vi "Refresh Default Value.vi"(8 "error in (no error)":errorcluster, 10 "Label":T1, 11 "Param Ref in":T5 format="%.0x") -> (0 "error out":errorcluster, 3 "Param Ref out":T5 format="%.0x")   [LabVIEW 2012, in "AIT 429 System Explorer.lvlib"]
uses:
  AIT 429 System Explorer.lvlib
  <vilib>/NI Veristand/Custom Device API/Custom Device Item Ref.ctl
  Controls/AIT_Label.ctl
  Controls/AIT_Word.ctl
  Controls/ARINCParam.ctl
  Shared/Controls and Global/TransferType.ctl
  <vilib>/NI Veristand/Custom Device Tools/Custom Device Utility Library/NI VeriStand - Search for All Items by GUID.vi
  Shared/Controls and Global/Global.vi
  <vilib>/NI Veristand/Custom Device API/Get Item Property (Double).vi
  <vilib>/NI Veristand/Custom Device API/Get Item Property (I32).vi
  <vilib>/NI Veristand/Custom Device API/Get Item Property (Boolean).vi
  ARINC 429 Shared.lvlib
  <vilib>/NI Veristand/Custom Device API/Custom Device API.lvlib
  <vilib>/NI Veristand/Custom Device Tools/Custom Device Utility Library/Custom Device Utility Library.lvlib
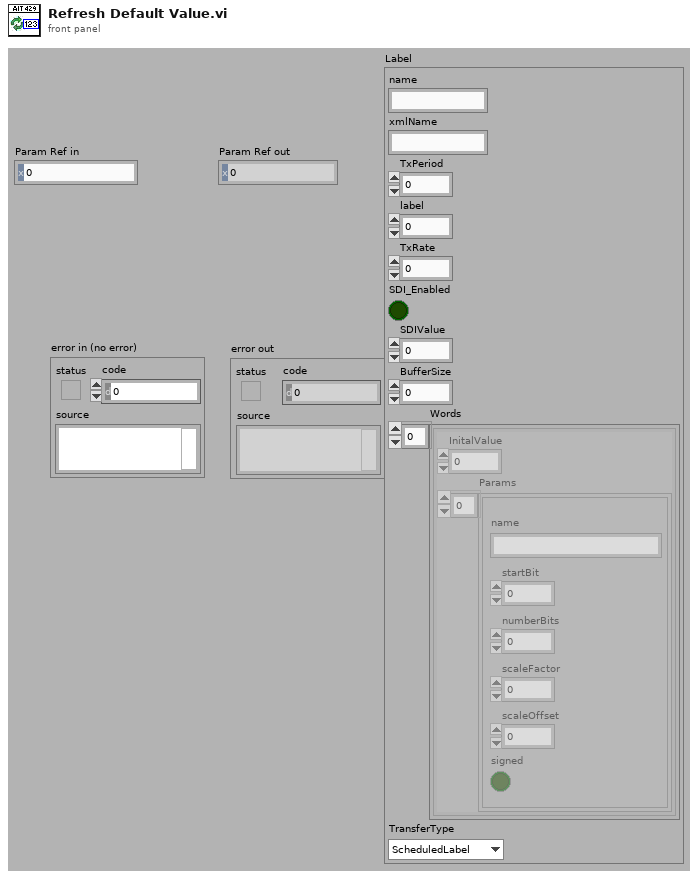
[diagram p1: front panel]
types:
  T1 = typedef "AIT 429 System Explorer.lvlib/AIT_Label.ctl" = cluster{"name":string, "xmlName":string, "TxPeriod":u32, "label":u32, "TxRate":dbl, "SDI_Enabled":bool, "SDIValue":u8, "BufferSize":u32, "Words":T2[], "TransferType":T4}
  T2 = typedef "AIT 429 System Explorer.lvlib/AIT_Word.ctl" = cluster{"InitalValue":u32, "Params":T3[]}
  T3 = typedef "AIT 429 System Explorer.lvlib/ARINCParam.ctl" = cluster{"name":string, "startBit":i32, "numberBits":i32, "scaleFactor":dbl, "scaleOffset":dbl, "signed":bool}
  T4 = typedef "ARINC 429 Shared.lvlib/TransferType.ctl" = enum16{"ScheduledLabel", "Acyclic", "Block", "Strobe"}
  T5 = typedef "Custom Device API.lvlib/Custom Device Item Ref.ctl" = u64
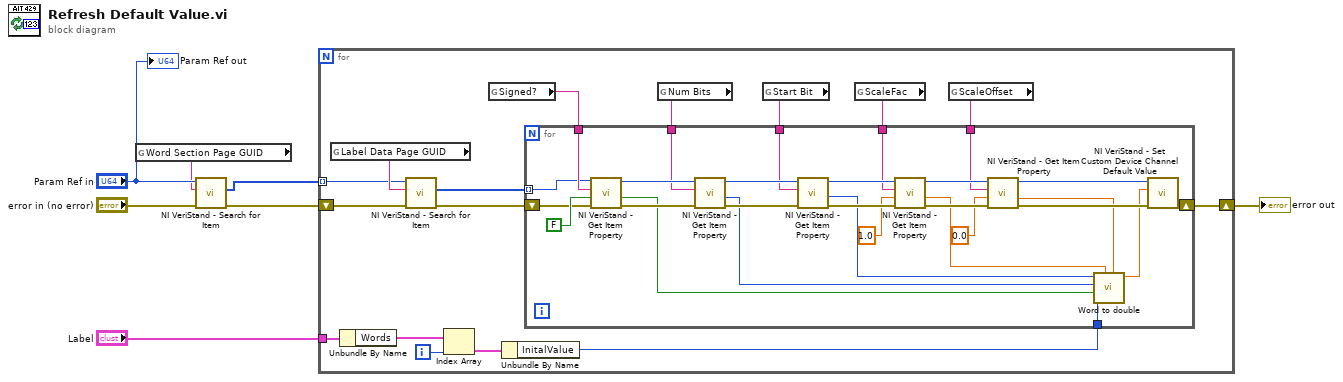
[diagram p0: block diagram]
diagram:
  n1 = global read "Global.vi" "Word Section Page GUID"() -> (w3:string)
  n2 = call-poly <vilib>:"NI VeriStand - Search for Item.vi"("error in"="error in (no error)", "Item GUID"=w3, "Section Ref in"="Param Ref in") -> ("error out"=w5:errorcluster, "Item Refs"=w2:T5[])  [unwired: 5 in, 2 out]
  n3 = for {
    shift-right: [w18] -> w7
    shift-left: w5 -> [w14]
    tunnel: w2 -> [w13] mode=indexing
    tunnel: "Label" -> [w12]
    i -> [w10]
    n4 = global read "Global.vi" "Label Data Page GUID"() -> (w17:string)
    n5 = Unbundle By Name(w12) -> ("Words"=w11:T2[])
    n6 = call-poly <vilib>:"NI VeriStand - Search for Item.vi"("error in"=w14, "Item GUID"=w17, "Section Ref in"=w13) -> ("error out"=w16:errorcluster, "Item Refs"=w15:T5[])  [unwired: 5 in, 2 out]
    n7 = Index Array(array=w11, index=w10) -> (element=w9:T2)
    n8 = global read "Global.vi" "Signed?"() -> (w23:string)
    n9 = Unbundle By Name(w9) -> ("InitalValue"=w8:u32)
    n10 = global read "Global.vi" "Num Bits"() -> (w22:string)
    n11 = global read "Global.vi" "Start Bit"() -> (w21:string)
    n12 = global read "Global.vi" "ScaleFac"() -> (w20:string)
    n13 = global read "Global.vi" "ScaleOffset"() -> (w19:string)
    n14 = for {
      tunnel: w8 -> [w51]
      tunnel: w23 -> [w50]
      tunnel: w22 -> [w46]
      tunnel: w21 -> [w43]
      tunnel: w20 -> [w38]
      tunnel: w19 -> [w35]
      shift-right: [w32] -> w18
      shift-left: w16 -> [w24]
      tunnel: w15 -> [w25] mode=indexing
      n15 = call-poly <vilib>:"NI VeriStand - Get Item Property.vi"("error in (no error)"=w24, "Default Value"=FALSE, "Property Name"=w50, "Item Ref in"=w25) -> ("error out"=w49:errorcluster, "Value"=w26:bool, "Item Ref out"=w48:T5)  [unwired: 4 in, 1 out]
      n16 = call-poly <vilib>:"NI VeriStand - Get Item Property.vi"("error in (no error)"=w49, "Property Name"=w46, "Item Ref in"=w48) -> ("error out"=w45:errorcluster, "Value"=w27:i32, "Item Ref out"=w44:T5)  [unwired: 5 in, 1 out]
      n17 = call-poly <vilib>:"NI VeriStand - Get Item Property.vi"("error in (no error)"=w45, "Property Name"=w43, "Item Ref in"=w44) -> ("error out"=w42:errorcluster, "Value"=w28:i32, "Item Ref out"=w41:T5)  [unwired: 5 in, 1 out]
      n18 = call-poly <vilib>:"NI VeriStand - Get Item Property.vi"("error in (no error)"=w42, "Default Value"=1.0 ("Scale Factor"), "Property Name"=w38, "Item Ref in"=w41) -> ("error out"=w39:errorcluster, "Value"=w29:dbl, "Item Ref out"=w40:T5)  [unwired: 4 in, 1 out]
      n19 = call-poly <vilib>:"NI VeriStand - Get Item Property.vi"("error in (no error)"=w39, "Default Value"=0.0 ("Scale Factor"), "Property Name"=w35, "Item Ref in"=w40) -> ("error out"=w34:errorcluster, "Value"=w30:dbl, "Item Ref out"=w33:T5)  [unwired: 4 in, 1 out]
      n20 = call "Word to double.vi"("ScaleOffset (0)"=w30, "ScaleFac (1)"=w29, "word"=w51, "Signed? (F)"=w26, "Number of Bits"=w27, "Start Bit"=w28) -> ("Double"=w31:dbl)  [unwired: 5 in]
      n21 = call <vilib>:"NI VeriStand - Set Custom Device Channel Default Value.vi"("error in (no error)"=w34, "Default Value"=w31, "Channel Ref in"=w33) -> ("error out"=w32:errorcluster)  [unwired: 7 in, 1 out]
    }
  }
  "error out" <- w7
  "Param Ref out" <- "Param Ref in"
